vi "RunLoadSummary1.vi"() -> ()   [LabVIEW 2012]
uses:
  Global1.vi
  <vilib>/Utility/file.llb/Read From Spreadsheet File (string).vi
  <vilib>/regexp/Match Regular Expression.xnode
panel:
  out "error out 2":errorcluster
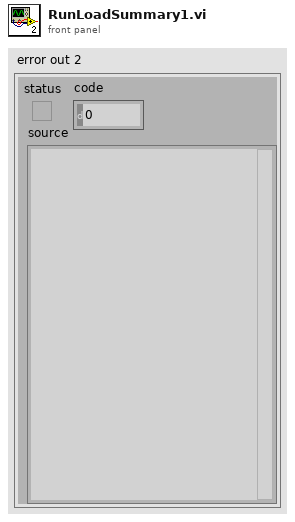
[diagram p1: front panel]
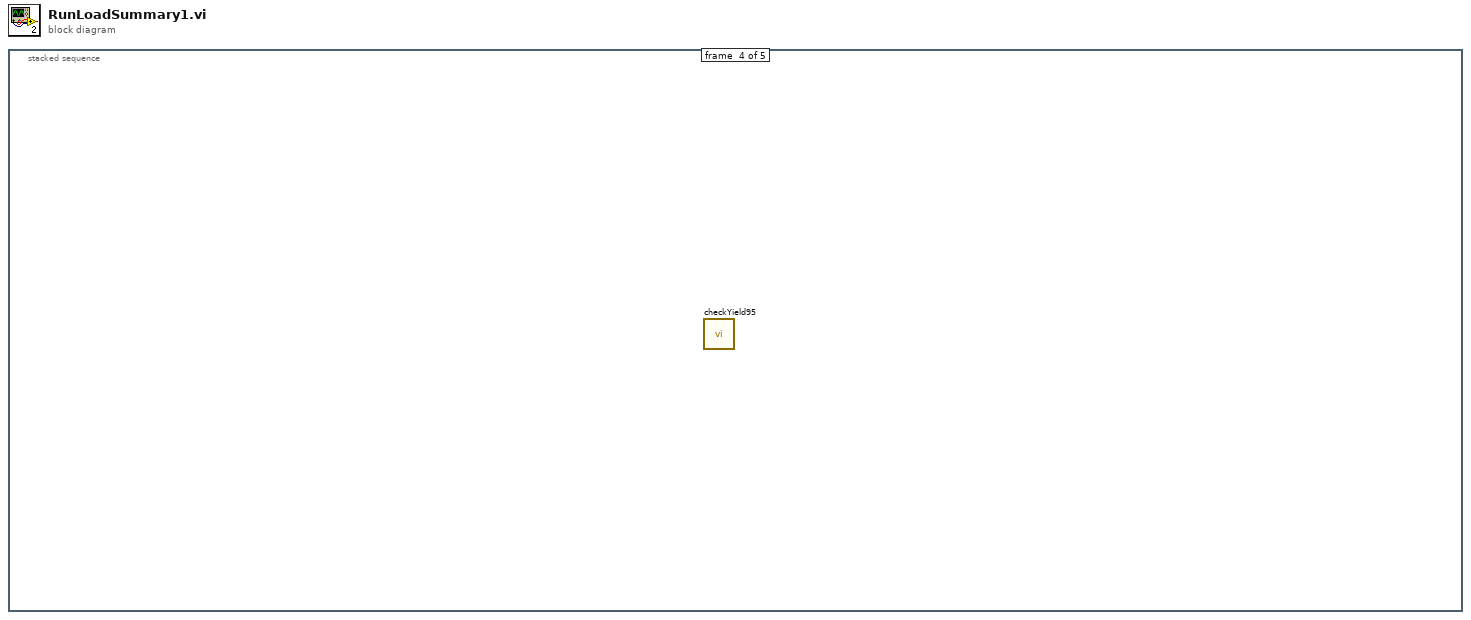
[diagram p0: block diagram]
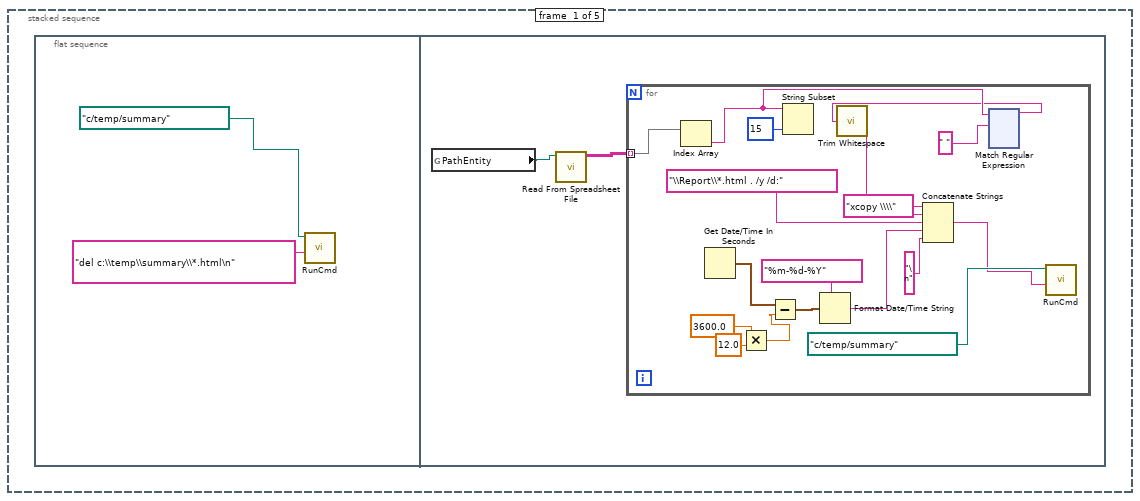
[diagram p2: hidden frame]
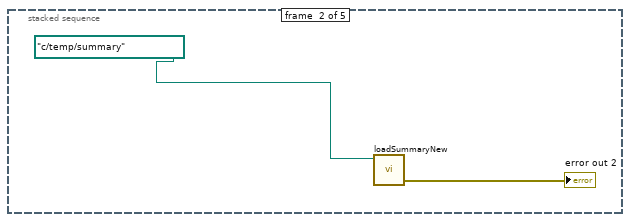
[diagram p3: hidden frame]
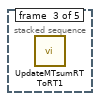
[diagram p4: hidden frame]
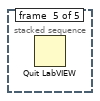
[diagram p5: hidden frame]
diagram:
  n1 = stacked-sequence {
    frame #0 {
      n2 = flat-sequence {
        frame #0 {
          n3 = call "RunCmd.vi"("Cmd String"="del c:\\temp\\summary\\*.html\n", "working directory"=path "c:/temp/summary") -> ()  [unwired: 8 in, 2 out]
        }
        frame #1 {
          n4 = global read "Global1.vi" "PathEntity"() -> (w3:path)
          n5 = call-poly <vilib>:"Read From Spreadsheet File.vi"("file path (dialog if empty)"=w3) -> ("all rows"=w4:string[][])  [unwired: 6 in, 4 out]
          n6 = for {
            tunnel: w4 -> [w8] mode=indexing
            n7 = Index Array(array=w8) -> (element=w6:string)  [unwired: 1 in]
            n8 = Get Date/Time In Seconds() -> (seconds since 1Jan1904=w15:timestamp)
            n9 = Multiply(x=3600.0, y=12.0) -> (x*y=w17:dbl)
            n10 = Subtract(x=w15, y=w17) -> (x-y=w18:timestamp)
            n11 = String Subset(string=w6, length (rest)=15 ("length (rest)")) -> ()  [unwired: 1 in, 1 out]
            n12 = Format Date/Time String(time format string (%c)="%m-%d-%Y", seconds (now)=w18) -> (date/time string=w20:string)  [unwired: 1 in]
            n13 = xnode "Match Regular Expression"("input string"=w6, "regular expression"=" ") -> ("before match"=w5:string)  [unwired: 4 in, 4 out]
            n14 = call <vilib>:"Trim Whitespace.vi"("string"=w5) -> ("trimmed string"=w9:string)  [unwired: 1 in]
            n15 = Concatenate Strings("xcopy \\\\" ("string"), w9, "\\Report\\*.html . /y /d:" ("string"), w20, "\n" ("string")) -> (w11:string)
            n16 = call "RunCmd.vi"("Cmd String"=w11, "working directory"=path "c:/temp/summary") -> ()  [unwired: 8 in, 2 out]
          }
        }
      }
    }
    frame #1 {
      n17 = call "loadSummaryNew.vi"("path"=path "c:/temp/summary" ("working directory")) -> ("error out"=→"error out 2":errorcluster)  [unwired: 10 in]
    }
    frame #2 {
      n18 = call "UpdateMTsumRTToRT1.vi"() -> ()  [unwired: 12 in]
    }
    frame #3 {
      n19 = call "checkYield95.vi"() -> ()  [unwired: 12 in]
    }
    frame #4 {
      n20 = Quit LabVIEW() -> ()  [unwired: 1 in]
    }
  }
